vi "Delay Timer.vi"(4 "error in":errorcluster, 7 "milliseconds to wait":u32) -> (0 "error out":errorcluster)   [LabVIEW 2014]
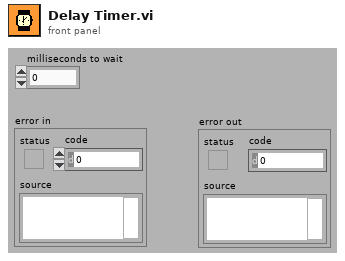
[diagram p1: front panel]
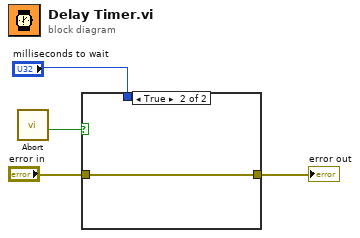
[diagram p0: block diagram]
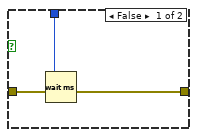
[diagram p2: hidden frame]
diagram:
  n1 = call "Abort.vi"() -> ("Abort out"=w1:bool)  [unwired: 7 in, 1 out]
  n2 = case shown="True" w1 {
    tunnel: "milliseconds to wait" -> [w6 _]
    tunnel: [w5 w7] -> w3
    tunnel: "error in" -> [w5 w7]
    frame False {
      n3 = Wait (ms)(milliseconds to wait=w6) -> ()  [unwired: 1 out]
    }
    frame True {
    }
  }
  "error out" <- w3
